vi "TX_logic.vi"(5 "Settings":T1, 9 "TX_data":u16) -> (4 "Busy":bool, 6 "TX":bool)   [LabVIEW 2015, in "UART_Firmware.lvlib"]
uses:
  UART_Firmware.lvlib
  Settings.ctl
  Parity.ctl
  StopBits.ctl
  TX_State.ctl
  TX_State_Data.ctl
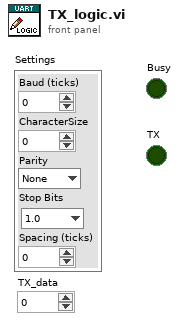
[diagram p1: front panel]
types:
  T1 = typedef "UART_Firmware.lvlib/Settings.ctl" = cluster{"Baud (ticks)":u32, "CharacterSize":u8, "Parity":T2, "Stop Bits":T3, "Spacing (ticks)":u32}
  T2 = typedef "UART_Firmware.lvlib/Parity.ctl" = enum8{"None", "Even", "Odd"}
  T3 = typedef "UART_Firmware.lvlib/StopBits.ctl" = enum8{"1.0", "1.5", "2.0"}
  T4 = typedef "UART_Firmware.lvlib/TX_State.ctl" = enum8{"Idle", "Start", "Character", "Parity", "Stop", "CharSpacing"}
  T5 = typedef "UART_Firmware.lvlib/TX_State_Data.ctl" = cluster{"Character":u16, "CharCount":u8, "Parity":bool}
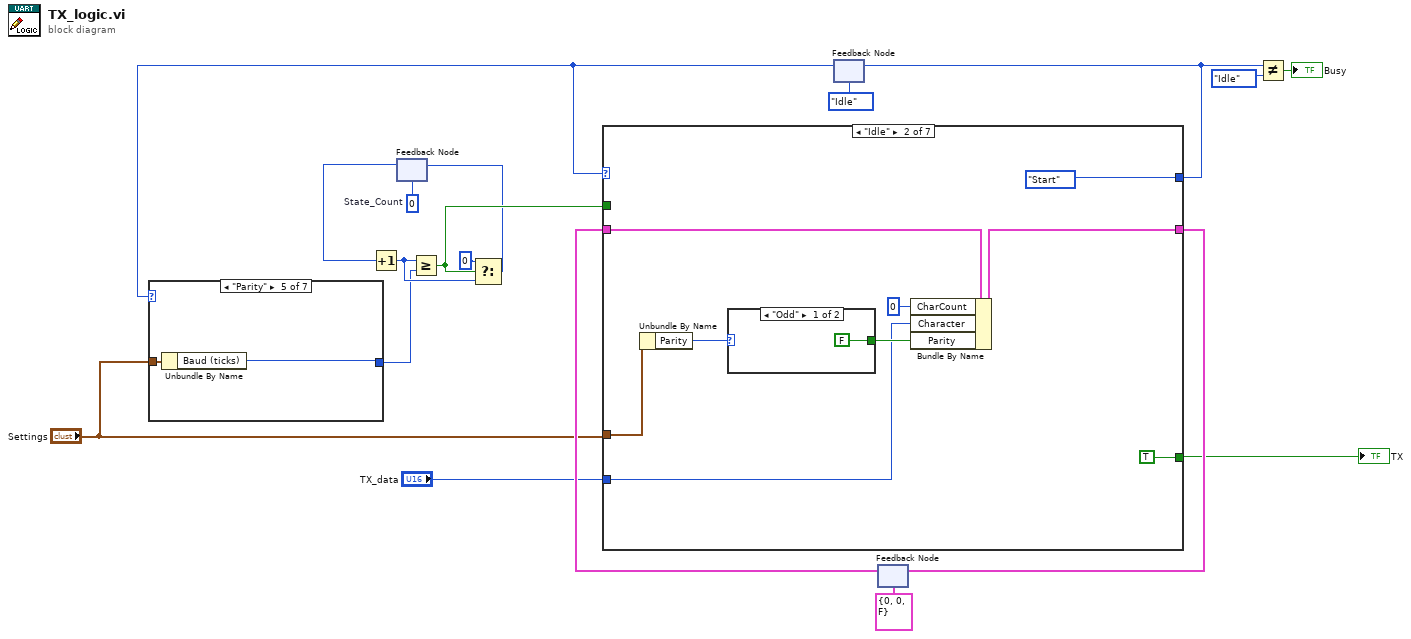
[diagram p0: block diagram]
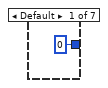
[diagram p2: hidden frame]
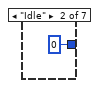
[diagram p3: hidden frame]
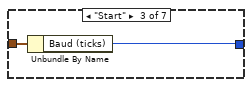
[diagram p4: hidden frame]
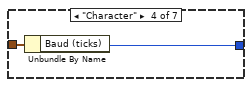
[diagram p5: hidden frame]
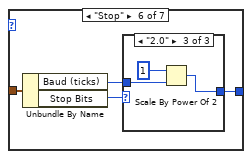
[diagram p6: hidden frame]
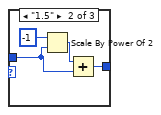
[diagram p8: hidden frame]
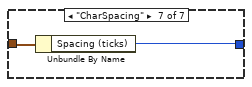
[diagram p9: hidden frame]
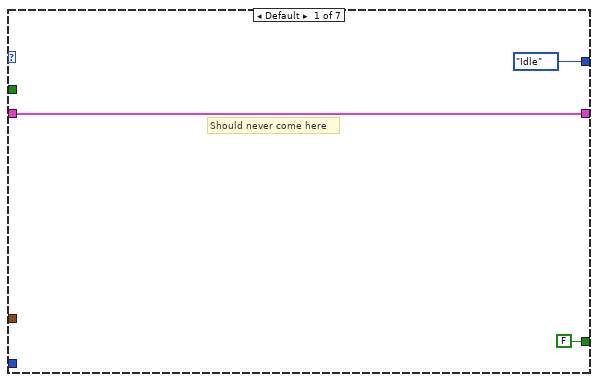
[diagram p10: hidden frame]
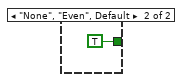
[diagram p11: hidden frame]
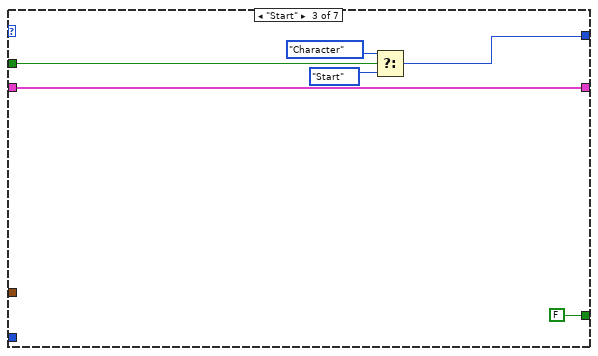
[diagram p12: hidden frame]
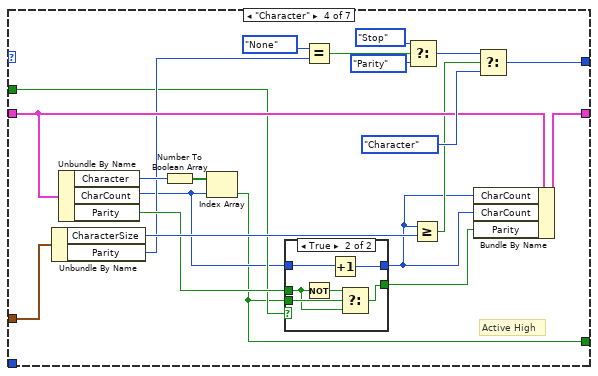
[diagram p13: hidden frame]
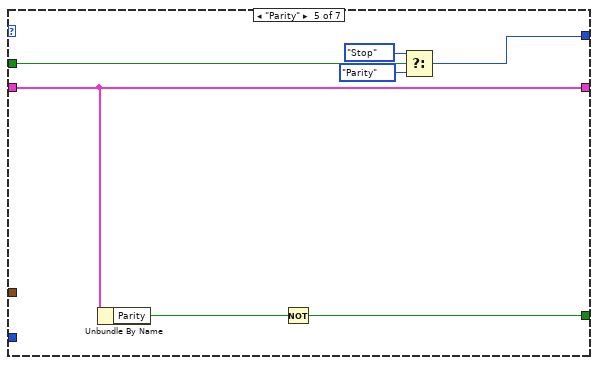
[diagram p15: hidden frame]
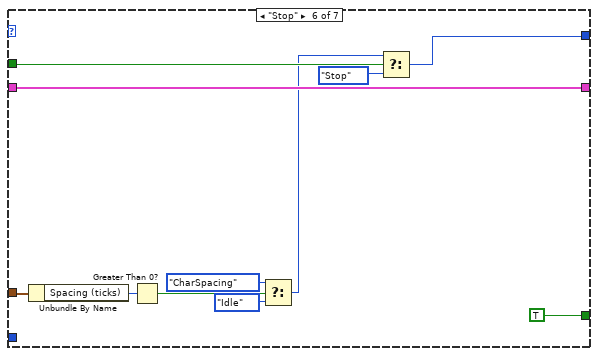
[diagram p16: hidden frame]
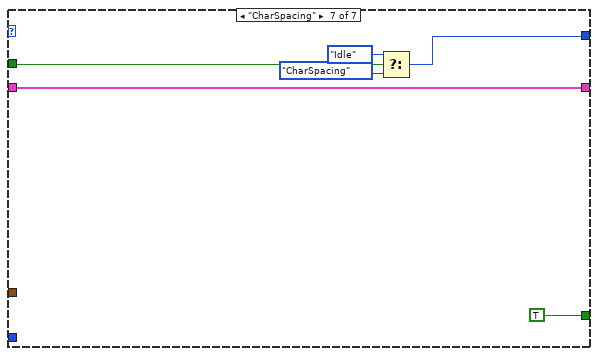
[diagram p17: hidden frame]
diagram:
  w7 = u32 0  # State_Count
  n1 = feedback #1(w7) -> (w6:u32)
  n2 = Increment(x=w6) -> (x+1=w11:u32)
  n3 = feedback #2(TX_State."Idle" ("TX State")) -> (w9:T4)
  n4 = case shown="\"Parity\"" w9 {
    tunnel: "Settings" -> [_ _ w22 w24 w26 w30 w40]
    tunnel: [u32 0 ("y") u32 0 ("y") w21 w23 w25 w27 w39] -> w8
    frame Default {
    }
    frame "Idle" {
    }
    frame "Start" {
      n5 = Unbundle By Name(w22) -> ("Baud (ticks)"=w21:u32)
    }
    frame "Character" {
      n6 = Unbundle By Name(w24) -> ("Baud (ticks)"=w23:u32)
    }
    frame "Parity" {
      n7 = Unbundle By Name(w26) -> ("Baud (ticks)"=w25:u32)
    }
    frame "Stop" {
      n8 = Unbundle By Name(w30) -> ("Baud (ticks)"=w28:u32, "Stop Bits"=w29:T3)
      n9 = case shown="\"2.0\"" w29 {
        tunnel: w28 -> [w31 w32 w38]
        tunnel: [w31 w34 w36] -> w27
        frame "1.0", Default {
        }
        frame "1.5" {
          n10 = Scale By Power Of 2(n=-1, x=w32) -> (x*2^n=w33:u32)
          n11 = Add(x=w33, y=w32) -> (x+y=w34:u32)
        }
        frame "2.0" {
          n12 = Scale By Power Of 2(n=1, x=w38) -> (x*2^n=w36:u32)
        }
      }
    }
    frame "CharSpacing" {
      n13 = Unbundle By Name(w40) -> ("Spacing (ticks)"=w39:u32)
    }
  }
  n14 = Greater Or Equal?(x=w11, y=w8) -> (x >= y?=w10:bool)
  n15 = Select(t=u32 0 ("State_Count"), s=w10, f=w11) -> (s? t:f=w5:u32)
  n16 = feedback-in #1(w5) -> ()
  n17 = feedback #3(T5 {"Character"=0, "CharCount"=0, "Parity"=FALSE} ("TX_State_Data")) -> (w4:T5)
  n18 = case shown="\"Idle\"" w9 {
    tunnel: w4 -> [w42 w45 w56 w78 w92 w106 w112]
    tunnel: [TX_State."Idle" ("y") TX_State."Start" ("TX State") w57 w80 w94 w101 w109] -> w14
    tunnel: "Settings" -> [_ w50 _ w77 _ w104 _]
    tunnel: [w42 w44 w56 w79 w92 w106 w112] -> w17
    tunnel: [FALSE TRUE FALSE w61 w90 TRUE TRUE] -> w16
    tunnel: w10 -> [_ _ w55 w65 w93 w105 w111]
    tunnel: "TX_data" -> [_ w47 _ _ _ _ _]
    frame Default {
      # "Should never come here"
    }
    frame "Idle" {
      n19 = Unbundle By Name(w50) -> ("Parity"=w49:T2)
      n20 = case shown="\"Odd\"" w49 {
        tunnel: [FALSE TRUE] -> w48
        frame "Odd" {
        }
        frame "None", "Even", Default {
        }
      }
      n21 = Bundle By Name(cluster=w45, "CharCount"=u8 0 ("PayloadCount"), "Character"=w47, "Parity"=w48) -> (w44:T5)
    }
    frame "Start" {
      n22 = Select(t=TX_State."Character" ("y"), s=w55, f=TX_State."Start" ("y")) -> (s? t:f=w57:T4)
    }
    frame "Character" {
      # "Active High"
      n23 = Unbundle By Name(w77) -> ("CharacterSize"=w74:u8, "Parity"=w71:T2)
      n24 = Unbundle By Name(w78) -> ("Character"=w76:u16, "CharCount"=w64:u8, "Parity"=w72:bool)
      n25 = Number To Boolean Array(number=w76) -> (Boolean array=w75:bool[])
      n26 = Index Array(array=w75, index=w64) -> (element=w61:bool)
      n27 = case shown="True" w65 {
        tunnel: w72 -> [w83 w87]
        tunnel: [w83 w86] -> w63
        tunnel: w61 -> [_ w89]
        tunnel: w64 -> [w82 w85]
        tunnel: [w82 w84] -> w62
        frame False {
        }
        frame True {
          n28 = Not(x=w87) -> (.not. x?=w88:bool)
          n29 = Increment(x=w85) -> (x+1=w84:u8)
          n30 = Select(t=w88, s=w89, f=w87) -> (s? t:f=w86:bool)
        }
      }
      n31 = Equal?(x=Parity."None", y=w71) -> (x = y?=w69:bool)
      n32 = Select(t=TX_State."Stop" ("y"), s=w69, f=TX_State."Parity" ("y")) -> (s? t:f=w66:T4)
      n33 = Greater Or Equal?(x=w62, y=w74) -> (x >= y?=w73:bool)
      n34 = Bundle By Name(cluster=w78, "CharCount"=w62, "CharCount"=w62, "Parity"=w63) -> (w79:T5)
      n35 = Select(t=w66, s=w73, f=TX_State."Character" ("y")) -> (s? t:f=w80:T4)
    }
    frame "Parity" {
      n36 = Unbundle By Name(w92) -> ("Parity"=w91:bool)
      n37 = Not(x=w91) -> (.not. x?=w90:bool)
      n38 = Select(t=TX_State."Stop" ("TX State"), s=w93, f=TX_State."Parity") -> (s? t:f=w94:T4)
    }
    frame "Stop" {
      n39 = Unbundle By Name(w104) -> ("Spacing (ticks)"=w103:u32)
      n40 = Greater Than 0?(x=w103) -> (x > 0?=w100:bool)
      n41 = Select(t=TX_State."CharSpacing" ("TX State"), s=w100, f=TX_State."Idle" ("TX State")) -> (s? t:f=w97:T4)
      n42 = Select(t=w97, s=w105, f=TX_State."Stop" ("TX State")) -> (s? t:f=w101:T4)
    }
    frame "CharSpacing" {
      n43 = Select(t=TX_State."Idle" ("TX State"), s=w111, f=TX_State."CharSpacing" ("TX State")) -> (s? t:f=w109:T4)
    }
  }
  "TX" <- w16
  n44 = feedback-in #2(w14) -> ()
  n45 = feedback-in #3(w17) -> ()
  n46 = Not Equal?(x=w14, y=TX_State."Idle") -> (x != y?=→"Busy":bool)
